vi "StringProbe.vi"() -> ()   [LabVIEW 2010]
panel:
  out "String":string
  in  "Probe":string
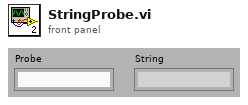
[diagram p1: front panel]
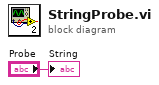
[diagram p0: block diagram]
diagram:
  "String" <- "Probe"
